vi "aft_xmpl_SNR.vi"(0 "Signal":dbl[](array[numeric]), 1 "Noise":dbl[](array[numeric])) -> (5 "snr":dbl)   [LabVIEW 2019]
uses:
  <vilib>/Analysis/baseanly.llb/Real Dot Product.vi
  <vilib>/Analysis/NI_AALBase.lvlib
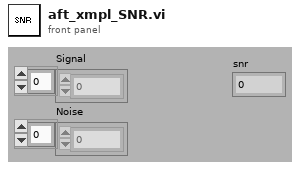
[diagram p1: front panel]
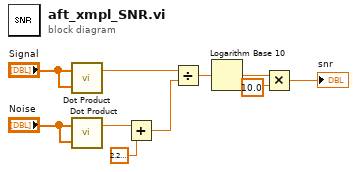
[diagram p0: block diagram]
diagram:
  n1 = call-poly <vilib>:"Dot Product.vi"("Y Vector"="Signal", "X Vector"="Signal") -> ("X * Y"=w10:dbl)  [unwired: 1 out]
  n2 = call-poly <vilib>:"Dot Product.vi"("Y Vector"="Noise", "X Vector"="Noise") -> ("X * Y"=w2:dbl)  [unwired: 1 out]
  n3 = Add(x=w2, y=2.220446049250313e-16) -> (x+y=w1:dbl)
  n4 = Divide(x=w10, y=w1) -> (x/y=w9:dbl)
  n5 = Logarithm Base 10(1:w9) -> (0:w8:dbl)
  n6 = Multiply(x=w8, y=10.0) -> (x*y=→"snr":dbl)
